vi "ReadSQLite.vi"(6 "Orden":string(combo)="ASC", 7 "Elemento":string(combo)="Torque", 8 "error in (no error)":errorcluster, 10 "Limit Control":i32=30, 11 "Path Control":path=path "C:/SQLite Data Bases/Project DB/Project.db") -> (0 "error in (no error) 3":errorcluster, 2 "Table":string[][](table))   [LabVIEW 2020]
doc: "This VI reads data from a SQLite DB"
uses:
  <vilib>/drjdpowell/SQLite Library/SQL Connection/Open (path).vi
  <vilib>/drjdpowell/SQLite Library/SQL Connection/Open (string).vi
  <vilib>/AdvancedString/Path To Command Line String.vi
  <vilib>/drjdpowell/SQLite Library/SQL Connection/Execute SQL.vi
  <vilib>/drjdpowell/SQLite Library/SQL Connection/Connection.lvclass
  <vilib>/drjdpowell/SQLite Library/SQLite.lvlib
panel:
  out "resulting string":string
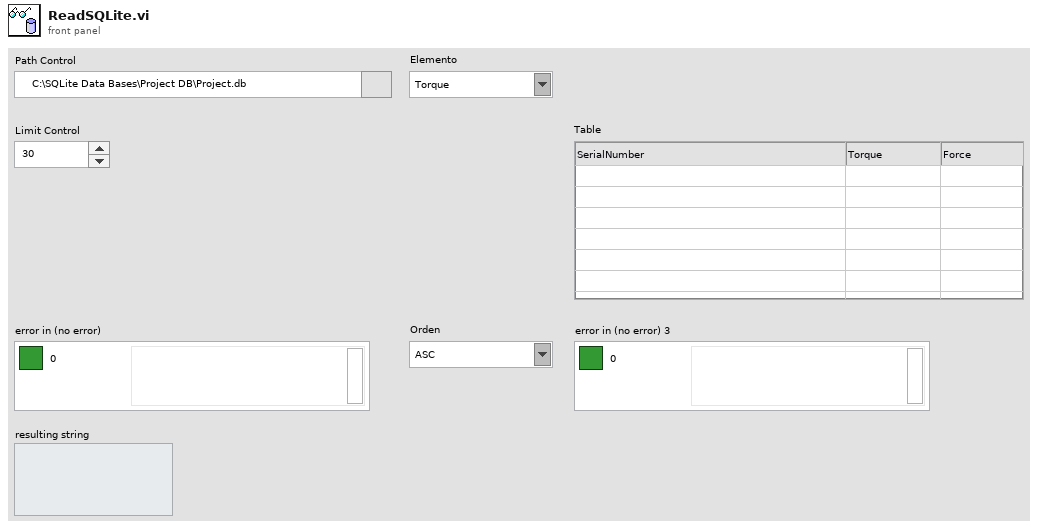
[diagram p1: front panel]
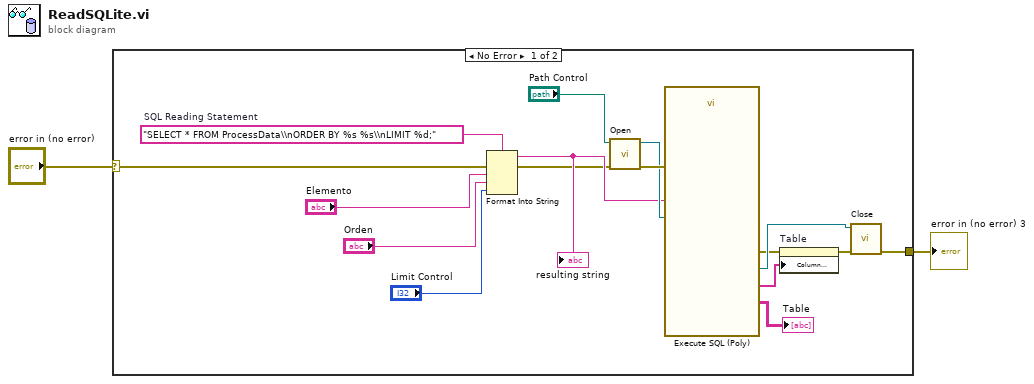
[diagram p0: block diagram]
diagram:
  n1 = case shown="No Error" "error in (no error)" {
    selector: "error in (no error)" -> [w4 w19]
    tunnel: [w14 w19] -> w1
    frame No Error {
      w9 = "SELECT * FROM ProcessData\\nORDER BY %s %s\\nLIMIT %d;"  # SQL Reading Statement
      n2 = Format Into String "Format Into String"(format string=w9, error in=w4, "Elemento", "Orden", "Limit Control") -> (resulting string=w8:string, error out=w3:errorcluster)  [unwired: 1 in]
      "resulting string" <- w8
      n3 = call-poly <vilib>:"Open.vi"("error in (no error)"=w3, "db file"="Path Control") -> ("error out"=w17:errorcluster, "SQLite Connection"=w15:refnum<class "Connection.lvclass">)  [unwired: 8 in]
      n4 = call-poly <vilib>:"Execute SQL (Poly).vi"("error in (no error)"=w17, "SQL"=w8, "SQLite Connection in"=w15) -> ("error out"=w11:errorcluster, "Column Names"=w12:string[], "Result Set"=→"Table":string[][], "SQLite Connection"=w16:refnum<class "Connection.lvclass">)  [unwired: 5 in]
      n5 = property on="Table" class="Tbl (strict)"(error in=w11, "Column Headers[]"=w12) -> (error out=w10:errorcluster)  [unwired: 1 in, 1 out]
      n6 = call-dynamic "Close.vi"("error in (no error)"=w10, "SQLite Connection in"=w16) -> ("error out"=w14:errorcluster)  [unwired: 9 in]
    }
    frame Error {
    }
  }
  "error in (no error) 3" <- w1
